vi "Append Block.vi"(10 "block in":u8[](array[numeric]) format="%02x", 11 "Hash Function in":refnum<class "NI_SHA-3.lvclass">) -> (3 "Hash Function out":refnum<class "NI_SHA-3.lvclass">)   [LabVIEW 2020, in "NI_SHA-3.lvclass"]
doc: "Feed a single block of data into the state array. This effectively executes a single \"absorbing\" iteration of the sponge function."
uses:
  <vilib>/security/Message Digest/SHA-3/NI_SHA-3.lvclass
  <vilib>/security/Message Digest/SHA-3/NI_SHA-3.lvclass/NI_SHA-3.ctl
  8da7a7e0-5a7e-3fc5-a8fa-aa546adce93f.vi
  8da7a7e0-5a7e-3fc5-a8fa-aa546adce93f.vi/314a9fc0-e363-3fd3-6eb3-345ebc10ed3f.vi
  <vilib>/security/Message Digest/SHA-3/Get Block Size.vi
  <vilib>/security/Message Digest/SHA-3/subVIs/Get Word Type.vi
  8da7a7e0-5a7e-3fc5-a8fa-aa546adce93f.vi/314a9fc0-e363-3fd3-6eb3-345ebc10ed3f.vi/fd99a990-3659-3fe1-140c-8b78c144ec3f.vi
  <vilib>/security/Message Digest/SHA-3/Get Block Size.vi/eb1e6525-3e01-40a8-a5c2-e849aaf68d04.vi
  <vilib>/security/Message Digest/SHA-3/Get Block Size.vi/eb1e6525-3e01-40a8-a5c2-e849aaf68d04.vi/00efce51-7697-47ef-971b-245e50795e7f.vi
  <vilib>/security/Message Digest/SHA-3/subVIs/Get Capacity.vi
  <vilib>/security/Message Digest/SHA-3/subVIs/XOR Input Block.vi
  <vilib>/security/Message Digest/SHA-3/subVIs/All Rounds.vi
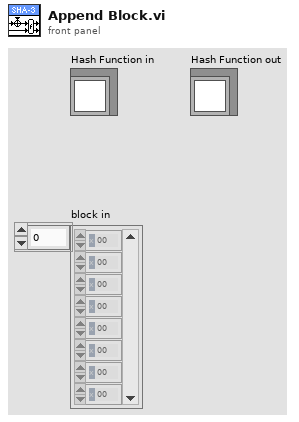
[diagram p1: front panel]
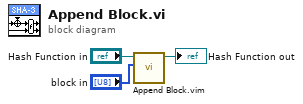
[diagram p0: block diagram]
diagram:
  n1 = call "Append Block.vim"("block in"="block in", "Hash Function in"="Hash Function in") -> ("Hash Function out"=→"Hash Function out":refnum<class "NI_SHA-3.lvclass">)  [unwired: 9 in]
